vi "Launcher (SubVI).vi"(8 "error in (no error)":errorcluster, 11 "String":string) -> (0 "error out":errorcluster, 3 "spreadsheet string":string)   [LabVIEW 2025]
uses:
  Full User Interface/Full User Interface.lvlib
  <vilib>/Utility/file.llb/Write Delimited Spreadsheet (string).vi
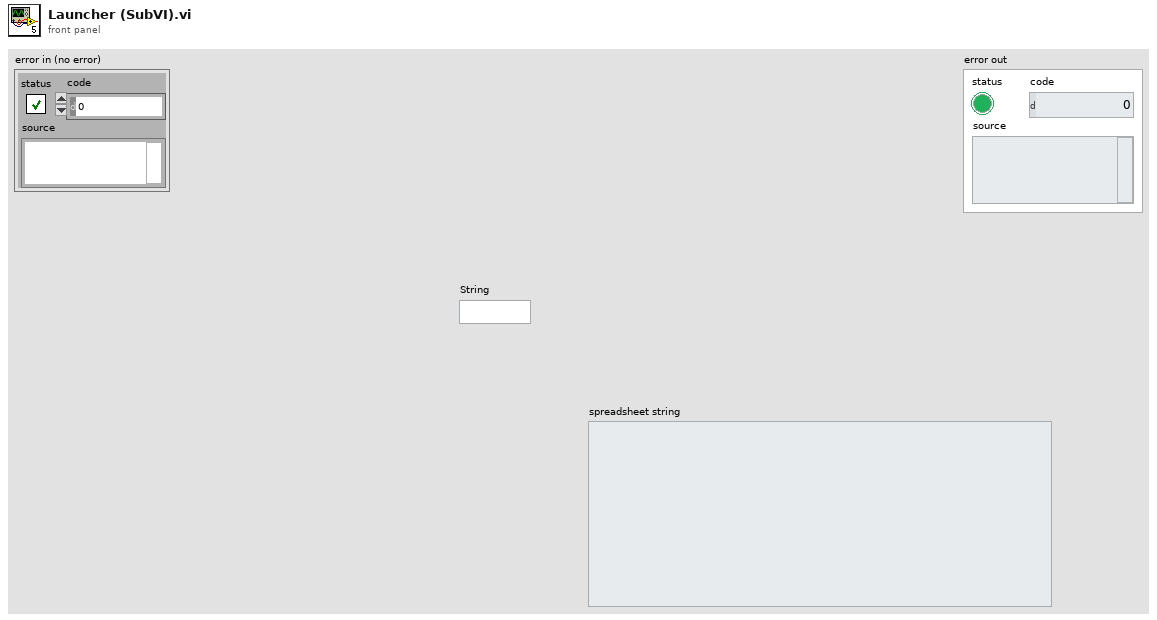
[diagram p1: front panel]
types:
  T1 = enum16{"open", "replace", "create", "open or create", "replace or create", "replace or create with confirmation"}
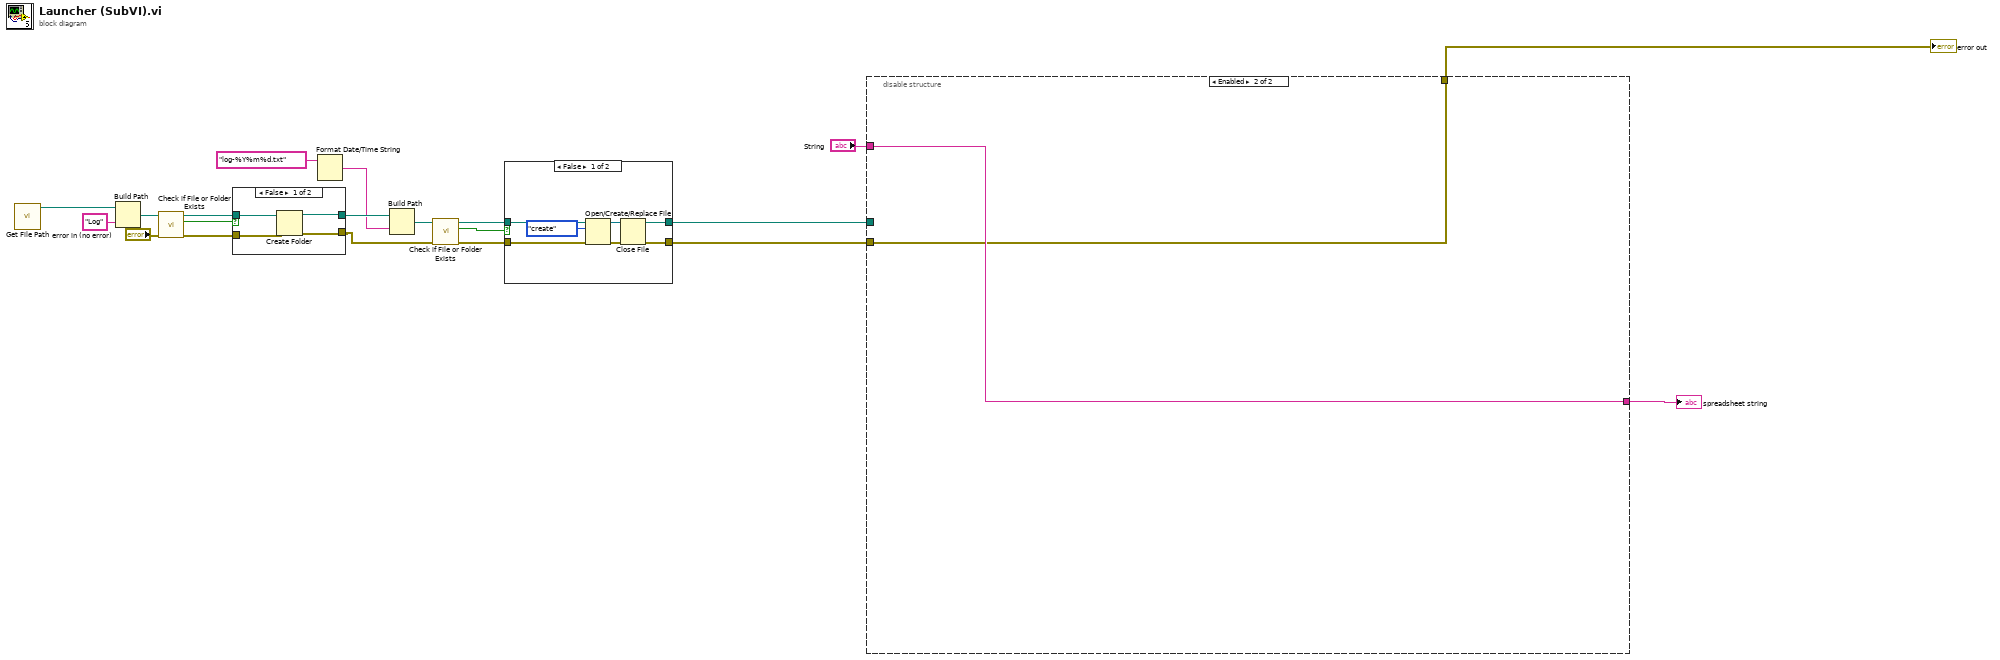
[diagram p0: block diagram]
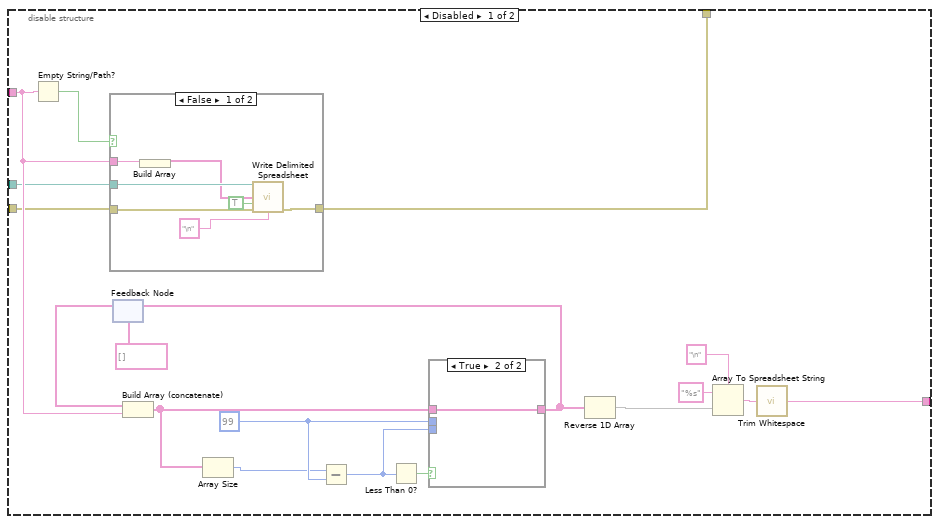
[diagram p2: hidden frame]
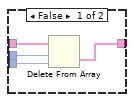
[diagram p3: hidden frame]
diagram:
  n1 = call "Get File Path.vi"() -> ("Application Directory"=w20:path)  [unwired: 11 in]
  n2 = Build Path(base path=w20, name or relative path="Log") -> (appended path=w17:path)
  n3 = call <vilib>:"Check if File or Folder Exists.vi"("error in (no error)"="error in (no error)", "path"=w17) -> ("error out"=w12:errorcluster, "file or folder exists?"=w16:bool, "dup path"=w15:path)  [unwired: 7 in]
  n4 = case shown="False" w16 {
    tunnel: w15 -> [w24 w26]
    tunnel: [w23 w26] -> w14
    tunnel: w12 -> [w22 w25]
    tunnel: [w21 w25] -> w7
    frame False {
      n5 = Create Folder(path (use dialog)=w24, error in=w22) -> (created path=w23:path, error out=w21:errorcluster)  [unwired: 1 in, 1 out]
    }
    frame True {
    }
  }
  n6 = Format Date/Time String(time format string (%c)="log-%Y%m%d.txt") -> (date/time string=w13:string)  [unwired: 2 in]
  n7 = Build Path(base path=w14, name or relative path=w13) -> (appended path=w8:path)
  n8 = call <vilib>:"Check if File or Folder Exists.vi"("error in (no error)"=w7, "path"=w8) -> ("error out"=w5:errorcluster, "file or folder exists?"=w4:bool, "dup path"=w6:path)  [unwired: 7 in]
  n9 = case shown="False" w4 {
    tunnel: [w30 w34] -> w1
    tunnel: [w29 w35] -> w2
    tunnel: w6 -> [w28 w35]
    tunnel: w5 -> [w27 w34]
    frame False {
      n10 = Open/Create/Replace File(file path (use dialog)=w28, error in=w27, operation (0:open)=T1."create") -> (refnum out=w31:refnum<file>, error out=w32:errorcluster)  [unwired: 3 in, 1 out]
      n11 = Close File(refnum=w31, error in=w32) -> (path=w29:path, error out=w30:errorcluster)
    }
    frame True {
    }
  }
  n12 = disable-structure shown="Enabled" {
    disable-tunnel: [w50 w68] -> w10
    disable-tunnel: [w49 w67] -> w9
    disable-tunnel: "String" -> [w42 w68]
    disable-tunnel: w2 -> [w39 _]
    disable-tunnel: w1 -> [w38 w67]
    frame Disabled {
      w47 = 99 ("length")
      n13 = Empty String/Path?(string/path=w42) -> (empty?=w48:bool)
      n14 = case shown="False" w48 {
        tunnel: w39 -> [w65 _]
        tunnel: w38 -> [w64 w66]
        tunnel: [w63 w66] -> w49
        tunnel: w42 -> [w62 _]
        frame False {
          n15 = Build Array(w62) -> (w61:string[])
          n16 = call-poly <vilib>:"Write Delimited Spreadsheet.vi"("file path (dialog if empty)"=w65, "1D data"=w61, "append to file? (new file:F)"=TRUE, "error in (no error)"=w64, "delimiter (\\t)"="\n" ("delimiter (\\t)")) -> ("error out"=w63:errorcluster)  [unwired: 9 in, 1 out]
        }
        frame True {
        }
      }
      n17 = feedback #1(string[] []) -> (w41:string[])
      n18 = Build Array (concatenate)(w41, w42) -> (w40:string[])
      n19 = Array Size(array=w40) -> (size(s)=w44:i32)
      n20 = Subtract(x=w44, y=w47) -> (x-y=w45:i32)
      n21 = Less Than 0?(x=w45) -> (x < 0?=w46:bool)
      n22 = case shown="True" w46 {
        tunnel: w40 -> [w57 w58]
        tunnel: w47 -> [w56 _]
        tunnel: [w54 w58] -> w37
        tunnel: w45 -> [w55 _]
        frame False {
          n23 = Delete From Array(array=w57, length=w56, index=w55) -> (deleted portion=w54:string[])  [unwired: 1 out]
        }
        frame True {
        }
      }
      n24 = feedback-in #1(w37) -> ()
      n25 = Reverse 1D Array(array=w37) -> (reversed array=w43:string[])
      n26 = Array To Spreadsheet String(delimiter (Tab)="\n", array=w43, 3:"%s" ("format string")) -> (spreadsheet string=w51:string)
      n27 = call <vilib>:"Trim Whitespace.vi"("string"=w51) -> ("trimmed string"=w50:string)  [unwired: 1 in]
    }
    frame Enabled {
    }
  }
  "spreadsheet string" <- w10
  "error out" <- w9
